vi "Stepper Motor Control.vi"() -> ()   [LabVIEW 2020]
uses:
  <vilib>/MakerHub/LINX/Public/Peripherals/Digital/Digital Write N Chans.vi
  <vilib>/MakerHub/LINX/Private/Local IO/LinxDigitalWrite.vi
  <vilib>/MakerHub/LINX/Public/Utilities/Check Channel.vi
  <vilib>/MakerHub/LINX/Public/Utilities/Open Serial.vi
  <vilib>/MakerHub/LINX/Private/Utilties/Generate Error.vi
  <vilib>/MakerHub/LINX/LMH-LINX.lvlib
panel:
  in  "Step Speed (ms)":u32(slide) max=100 step=10 scale=0.0..100.0
  in  "RCW":bool
  in  "RCCW":bool
  in  "CCW":bool
  in  "CW":bool
  in  "STOP":bool
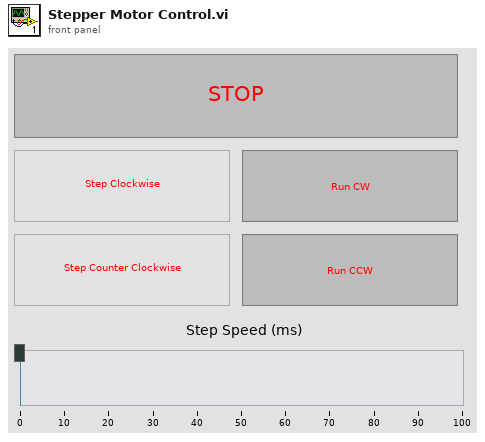
[diagram p1: front panel]
types:
  T1 = typedef "LMH-LINX.lvlib/LINX Ref.ctl" = cluster{"IO":T2, "Interface":T3, "LINX Device Config":T4}
  T2 = typedef "LMH-LINX.lvlib/Platform.ctl" = enum16{"Remote", "Local"}
  T3 = typedef "LMH-LINX.lvlib/Interface.ctl" = enum16{"Serial", "TCP"}
  T4 = typedef "LMH-LINX.lvlib/Device.lvlib/LINX Device Config.ctl" = cluster{"Interface":T3, "COM Port":refnum<visa-resource-name>, "TCP Configuration":T5, "Device Family":u8, "Device ID":u8, "Device Name":string, "TCP Ref":refnum<k5>, "Channels":T6}
  T5 = typedef "LMH-LINX.lvlib/Device.lvlib/TCP Config.ctl" = cluster{"IP Address":string, "Port":u16}
  T6 = typedef "LMH-LINX.lvlib/Channels.ctl" = cluster{"DI":u8[], "DO":u8[], "AI":u8[], "AO":u8[], "PWM":u8[], "QE":u8[], "UART":u8[], "I2C 2":u8[], "SPI":u8[], "CAN":u8[], "Servo":u8[], "AI Ref (V)":dbl, "AI Resolution (Bits)":u8, "AO Ref (V)":dbl, "AO Resolution (Bits)":u8}
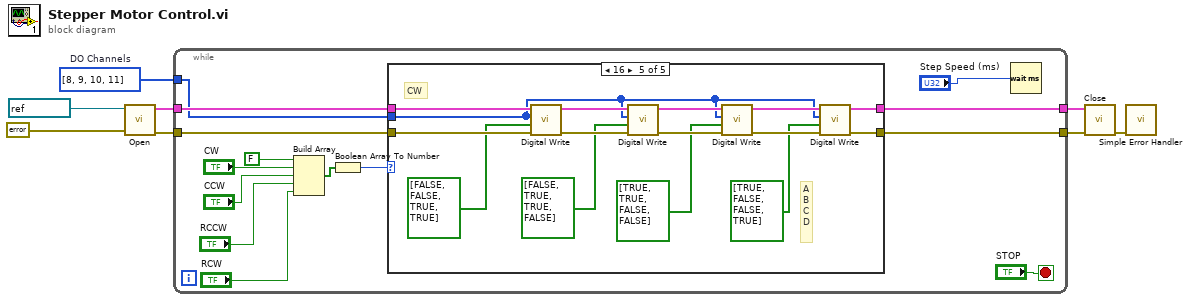
[diagram p0: block diagram]
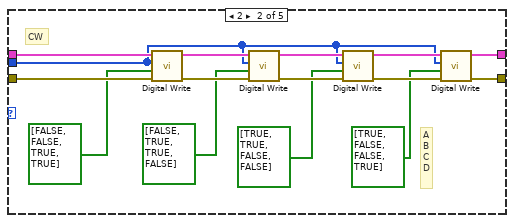
[diagram p3: hidden frame]
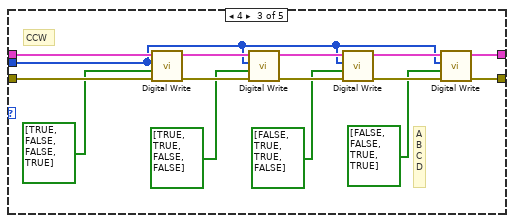
[diagram p4: hidden frame]
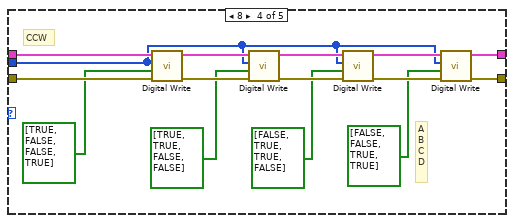
[diagram p5: hidden frame]
diagram:
  w2 = u8[] [8, 9, 10, 11]  # DO Channels
  n1 = call-poly <vilib>:"Open.vi"("Error In"=errorcluster {"status"=FALSE, "code"=0, "source"=""}, "Serial Port"=refnum<visa-resource-name> "COM5") -> ("Error Out"=w7:errorcluster, "LINX Resource"=w8:T1)  [unwired: 7 in, 1 out]
  n2 = while {
    tunnel: w8 -> [w21]
    tunnel: w7 -> [w20]
    tunnel: [w19] -> w4
    tunnel: [w18] -> w3
    tunnel: w2 -> [w17]
    stop <- "STOP" stop-if-true
    n3 = Build Array(FALSE ("Change Direction 2"), "CW", "CCW", "RCCW", "RCW") -> (w15:bool[])
    n4 = Boolean Array To Number(Boolean array=w15) -> (number=w14:u32)
    n5 = case shown="16" w14 {
      tunnel: w21 -> [w24 w39 w54 w69 w84]
      tunnel: w20 -> [w23 w38 w53 w68 w83]
      tunnel: [w24 w34 w49 w64 w79] -> w19
      tunnel: [w23 w33 w48 w63 w78] -> w18
      tunnel: w17 -> [_ w29 w44 w59 w74]
      frame 0, Default {
        # "do nothing"
      }
      frame 2 {
        # "A\nB\nC\nD"
        # "CW"
        n6 = call-poly <vilib>:"Digital Write.vi"("Error In"=w38, "Values"=bool[] [FALSE, FALSE, TRUE, TRUE], "DO Channels"=w29, "LINX Resource"=w39) -> ("Error Out"=w30:errorcluster, "LINX Resource"=w37:T1)  [unwired: 6 in]
        n7 = call-poly <vilib>:"Digital Write.vi"("Error In"=w30, "Values"=bool[] [FALSE, TRUE, TRUE, FALSE], "DO Channels"=w29, "LINX Resource"=w37) -> ("Error Out"=w31:errorcluster, "LINX Resource"=w36:T1)  [unwired: 6 in]
        n8 = call-poly <vilib>:"Digital Write.vi"("Error In"=w31, "Values"=bool[] [TRUE, TRUE, FALSE, FALSE], "DO Channels"=w29, "LINX Resource"=w36) -> ("Error Out"=w32:errorcluster, "LINX Resource"=w35:T1)  [unwired: 6 in]
        n9 = call-poly <vilib>:"Digital Write.vi"("Error In"=w32, "Values"=bool[] [TRUE, FALSE, FALSE, TRUE], "DO Channels"=w29, "LINX Resource"=w35) -> ("Error Out"=w33:errorcluster, "LINX Resource"=w34:T1)  [unwired: 6 in]
      }
      frame 4 {
        # "A\nB\nC\nD"
        # "CCW"
        n10 = call-poly <vilib>:"Digital Write.vi"("Error In"=w53, "Values"=bool[] [TRUE, FALSE, FALSE, TRUE], "DO Channels"=w44, "LINX Resource"=w54) -> ("Error Out"=w45:errorcluster, "LINX Resource"=w52:T1)  [unwired: 6 in]
        n11 = call-poly <vilib>:"Digital Write.vi"("Error In"=w45, "Values"=bool[] [TRUE, TRUE, FALSE, FALSE], "DO Channels"=w44, "LINX Resource"=w52) -> ("Error Out"=w46:errorcluster, "LINX Resource"=w51:T1)  [unwired: 6 in]
        n12 = call-poly <vilib>:"Digital Write.vi"("Error In"=w46, "Values"=bool[] [FALSE, TRUE, TRUE, FALSE], "DO Channels"=w44, "LINX Resource"=w51) -> ("Error Out"=w47:errorcluster, "LINX Resource"=w50:T1)  [unwired: 6 in]
        n13 = call-poly <vilib>:"Digital Write.vi"("Error In"=w47, "Values"=bool[] [FALSE, FALSE, TRUE, TRUE], "DO Channels"=w44, "LINX Resource"=w50) -> ("Error Out"=w48:errorcluster, "LINX Resource"=w49:T1)  [unwired: 6 in]
      }
      frame 8 {
        # "A\nB\nC\nD"
        # "CCW"
        n14 = call-poly <vilib>:"Digital Write.vi"("Error In"=w68, "Values"=bool[] [TRUE, FALSE, FALSE, TRUE], "DO Channels"=w59, "LINX Resource"=w69) -> ("Error Out"=w60:errorcluster, "LINX Resource"=w67:T1)  [unwired: 6 in]
        n15 = call-poly <vilib>:"Digital Write.vi"("Error In"=w60, "Values"=bool[] [TRUE, TRUE, FALSE, FALSE], "DO Channels"=w59, "LINX Resource"=w67) -> ("Error Out"=w61:errorcluster, "LINX Resource"=w66:T1)  [unwired: 6 in]
        n16 = call-poly <vilib>:"Digital Write.vi"("Error In"=w61, "Values"=bool[] [FALSE, TRUE, TRUE, FALSE], "DO Channels"=w59, "LINX Resource"=w66) -> ("Error Out"=w62:errorcluster, "LINX Resource"=w65:T1)  [unwired: 6 in]
        n17 = call-poly <vilib>:"Digital Write.vi"("Error In"=w62, "Values"=bool[] [FALSE, FALSE, TRUE, TRUE], "DO Channels"=w59, "LINX Resource"=w65) -> ("Error Out"=w63:errorcluster, "LINX Resource"=w64:T1)  [unwired: 6 in]
      }
      frame 16 {
        # "A\nB\nC\nD"
        # "CW"
        n18 = call-poly <vilib>:"Digital Write.vi"("Error In"=w83, "Values"=bool[] [FALSE, FALSE, TRUE, TRUE], "DO Channels"=w74, "LINX Resource"=w84) -> ("Error Out"=w75:errorcluster, "LINX Resource"=w82:T1)  [unwired: 6 in]
        n19 = call-poly <vilib>:"Digital Write.vi"("Error In"=w75, "Values"=bool[] [FALSE, TRUE, TRUE, FALSE], "DO Channels"=w74, "LINX Resource"=w82) -> ("Error Out"=w76:errorcluster, "LINX Resource"=w81:T1)  [unwired: 6 in]
        n20 = call-poly <vilib>:"Digital Write.vi"("Error In"=w76, "Values"=bool[] [TRUE, TRUE, FALSE, FALSE], "DO Channels"=w74, "LINX Resource"=w81) -> ("Error Out"=w77:errorcluster, "LINX Resource"=w80:T1)  [unwired: 6 in]
        n21 = call-poly <vilib>:"Digital Write.vi"("Error In"=w77, "Values"=bool[] [TRUE, FALSE, FALSE, TRUE], "DO Channels"=w74, "LINX Resource"=w80) -> ("Error Out"=w78:errorcluster, "LINX Resource"=w79:T1)  [unwired: 6 in]
      }
    }
    n22 = Wait (ms)(milliseconds to wait="Step Speed (ms)") -> ()  [unwired: 1 out]
  }
  n23 = call <vilib>:"Close.vi"("Error In"=w3, "LINX Resource"=w4) -> ("Error Out"=w1:errorcluster)  [unwired: 9 in]
  n24 = call <vilib>:"Simple Error Handler.vi"("error in (no error)"=w1) -> ()  [unwired: 4 in, 5 out]
